vi "gaussianGuesses.vi"(10 "X Values":dbl[](array[numeric]), 11 "Y Values":dbl[](array[numeric])) -> (2 "Guesses":dbl[](array[numeric]) caption="Initial Gaussian Fit Guesses")   [LabVIEW 2011]
uses:
  GaussianGlobal.vi
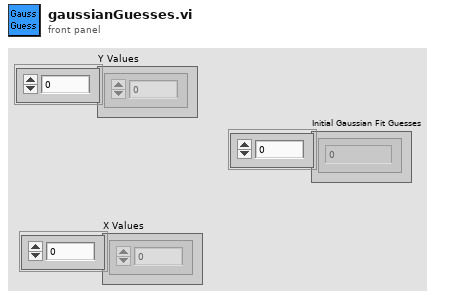
[diagram p1: front panel]
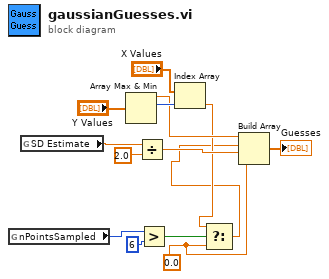
[diagram p0: block diagram]
diagram:
  w1 = 0.0 ("element")
  n1 = global read "GaussianGlobal.vi" "nPointsSampled"() -> (w6:i32)
  n2 = global read "GaussianGlobal.vi" "SD Estimate"() -> (w9:dbl)
  n3 = Array Max & Min(array="Y Values") -> (max value=w10:dbl, max index (indices)=w11:i32)  [unwired: 2 out]
  n4 = Divide(x=w9, y=2.0) -> (x/y=w7:dbl)
  n5 = Greater?(x=w6, y=6) -> (0:w4:bool)
  n6 = Index Array(array="X Values", index=w11) -> (element=w3:dbl)
  n7 = Select(t=w3, s=w4, f=w1) -> (s? t:f=w2:dbl)
  n8 = Build Array(w10, w2, w7, w1) -> (→"Guesses":dbl[])
